vi "Example Modbus Slave - ModbusSlaveWriteSingleRegisterRequestCallback Callback.vi"(4 "ModbusSlaveWriteSingleRegisterRequestCallback":refnum<user-event>, 5 "Event Data":T1, 6 "Control Ref":refnum<k24>, 7 "Event Common Data":T2) -> ()   [LabVIEW 2010]
uses:
  C:/tf/play/labview/Tinkerforge.dll
  Tinkerforge.dll
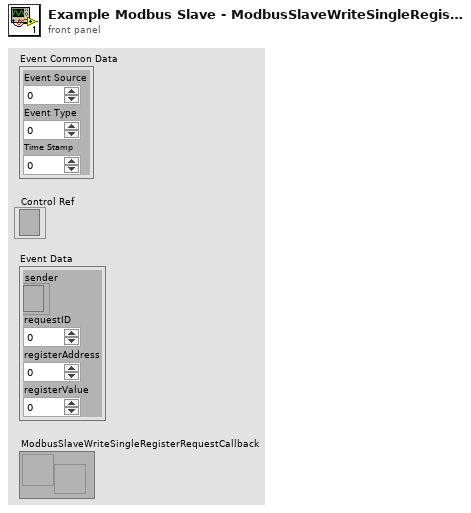
[diagram p1: front panel]
types:
  T1 = cluster{"sender":refnum<k24>, "requestID":u8, "registerAddress":i64, "registerValue":i32}
  T2 = cluster{"Event Source":i32, "Event Type":u32, "Time Stamp":u32}
  T3 = cluster{"requestID":u8, "registerAddress":i64, "registerValue":i32}
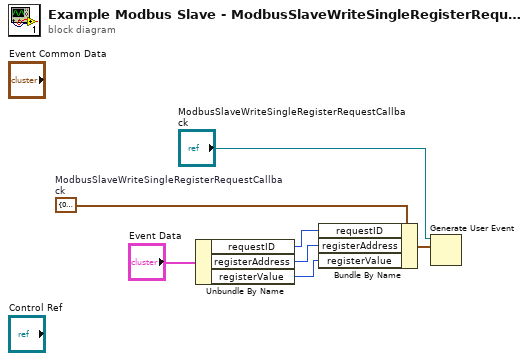
[diagram p0: block diagram]
diagram:
  w6 = T3 {"requestID"=0, "registerAddress"=0, "registerValue"=0}  # ModbusSlaveWriteSingleRegisterRequestCallback
  n1 = Unbundle By Name("Event Data") -> ("requestID"=w5:u8, "registerAddress"=w4:i64, "registerValue"=w3:i32)
  n2 = Bundle By Name(cluster=w6, "requestID"=w5, "registerAddress"=w4, "registerValue"=w3) -> (w2:T3)
  n3 = Generate User Event(user event="ModbusSlaveWriteSingleRegisterRequestCallback", event data cluster=w2) -> ()  [unwired: 1 in, 2 out]
